vi "Pre Launch Init.vi"(11 "RPI.SenseHat.Actor in":refnum<class "RPI.SenseHat.Actor.lvclass">) -> (0 "error out":errorcluster, 3 "RPI.SenseHat.Actor out":refnum<class "RPI.SenseHat.Actor.lvclass">)   [LabVIEW 2020, in "RPI.SenseHat.Actor.lvlib" / "RPI.SenseHat.Actor.lvclass"]
doc: "(<B>Filename</B>: Actor Framework.lvlib:Actor.lvclass:Pre Launch Init.vi)\n\nDefines behavior that occurs after the Launch Nested Actor method is invoked but before the actor's Actor Core method begins running.\n\nBy default, this method does nothing. A descendant class may override it to define behavior."
uses:
  RPI.SenseHat.Actor.lvclass
  C:/Program Files (x86)/National Instruments/LabVIEW 2020/vi.lib/ActorFramework/Actor/Actor.lvclass
  <vilib>/ActorFramework/Actor/Actor.lvclass/Actor.ctl
  <vilib>/ActorFramework/Message Enqueuer/Message Enqueuer.lvclass/Message Enqueuer.ctl
  <vilib>/ActorFramework/Message Enqueuer/Enqueue.vi
  <vilib>/ActorFramework/Message Enqueuer/Init from Existing Queue.vi
  RPI.SenseHat.Actor Messages/RPI.SenseHat Init Msg/RPI.SenseHat Init Msg.lvclass
  C:/Program Files (x86)/National Instruments/LabVIEW 2020/vi.lib/ActorFramework/Message/Message.lvclass
  <vilib>/ActorFramework/Message Priority Queue/Priority Enqueue.vi
  <vilib>/ActorFramework/Message Enqueuer/Message Enqueuer.lvclass
  <vilib>/ActorFramework/Actor/Actor.lvclass
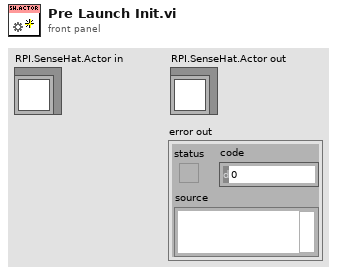
[diagram p1: front panel]
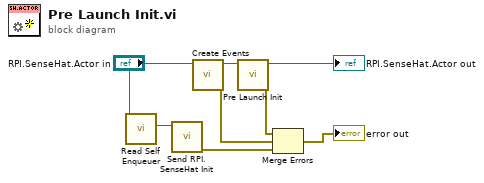
[diagram p0: block diagram]
diagram:
  n1 = call <vilib>:"Read Self Enqueuer.vi"("Actor"="RPI.SenseHat.Actor in") -> ("Self Enqueuer"=w3:refnum<class "Message Enqueuer.lvclass">)  [unwired: 10 in]
  n2 = call "Send RPI.SenseHat Init.vi"("Message Enqueuer"=w3) -> ("error out"=w1:errorcluster)  [unwired: 9 in, 1 out]
  n3 = call "Create Events.vi"("RPI.SenseHat.Actor in"="RPI.SenseHat.Actor in") -> ("error out"=w4:errorcluster, "RPI.SenseHat.Actor out"=w6:refnum<class "RPI.SenseHat.Actor.lvclass">)  [unwired: 9 in]
  n4 = call-parent "Pre Launch Init.vi"("Actor in"=w6) -> ("error out"=w8:errorcluster, "Actor out"=→"RPI.SenseHat.Actor out":refnum<class "RPI.SenseHat.Actor.lvclass">)  [unwired: 9 in]
  n5 = Merge Errors(w8, w4, w1) -> (→"error out":errorcluster)
